vi "testIFw.vi"() -> ()   [LabVIEW 2017]
uses:
  AFE/PI_Settings.ctl
  <vilib>/rvi/Analysis/control/PID/Typedef/niFpgaPID_PIGains.ctl
  <vilib>/rvi/Analysis/control/PID/Typedef/niFpgaPID_OutputRange.ctl
  AFE/Parameters.ctl
  AFE/Mode.ctl
  <instrlib>/_niInstr/FIFO Register Bus/v1/Host/niInstr FIFO Register Bus v1 Host.lvclass
  C:/Program Files (x86)/National Instruments/LabVIEW 2017/instr.lib/_niInstr/Instruction Framework/v1/Host/Instruction Target/niInstr Instruction Target v1 Host.lvclass
  <vilib>/FPGAPlugInAG/sbRIO-9607/niLvFpga_Open_sbRIO-9607.vi
  <vilib>/rvi/interface/common/dynamic/niFpgaDynamicAddResources.vi
  <vilib>/FPGAPlugInAG/Dynamic/niLvFpga_Reset_Dynamic.vi
  <vilib>/FPGAPlugInAG/Dynamic/niLvFpga_Run_Dynamic.vi
  <vilib>/Utility/error.llb/Error Cluster From Error Code.vi
  <vilib>/rvi/errors/niLvFpgaAdjustHostInterfaceError.vi
  <vilib>/FPGAPlugInAG/Dynamic/niLvFpga_Close_Dynamic.vi
  <vilib>/rvi/interface/nirviOpenFPGA/nirviOpenFPGA.xnode
  FPGA Bitfiles/AFE_FPGATarget_IFwTest_t2qLRm+eTm8.lvbitx
  IFwTest.vi
  <vilib>/rvi/interface/nirviMethod/nirviMethod.xnode
  <vilib>/rvi/interface/nirviReadWriteControl/nirviReadWriteControl.xnode
  <vilib>/rvi/interface/nirviCloseFPGA/nirviCloseFPGA.xnode
  AFE_Interface/AFE_interface.lvlib
  AFE/ActiveFrontEnd.lvlib
  NiFpgaLv.dll
  <vilib>/rvi/interface/Simulation/niFpgaSimulationCallBeginRW.vi
panel:
  in  "IQ_to_VQ":T1={"gains"={"proportional gain"=11.0, "integral gain"=12.0}, "output range"={"output high (Inf)"=13.0, "output low (-Inf)"=14.0}, "PI_state"=enum."perturbance", "reset"=TRUE, "manual"=15.0} {"gains"."proportional gain" step=0.125}
  in  "ID_to_VD":T1={"gains"={"proportional gain"=6.0, "integral gain"=7.0}, "output range"={"output high (Inf)"=8.0, "output low (-Inf)"=9.0}, "PI_state"=enum."manual", "reset"=TRUE, "manual"=10.0} {"gains"."proportional gain" step=0.125}
  in  "VDCLinkToPower":T1={"gains"={"proportional gain"=1.0, "integral gain"=2.0}, "output range"={"output high (Inf)"=3.0, "output low (-Inf)"=4.0}, "PI_state"=enum."normal", "reset"=TRUE, "manual"=5.0} {"gains"."proportional gain" step=0.125}
  out "IQ_to_VQ_PISettings":T4
  out "ID_to_VD_PISettings":T4
  out "VDCLinkToP_PISettings":T4
  out "Parameters":T5
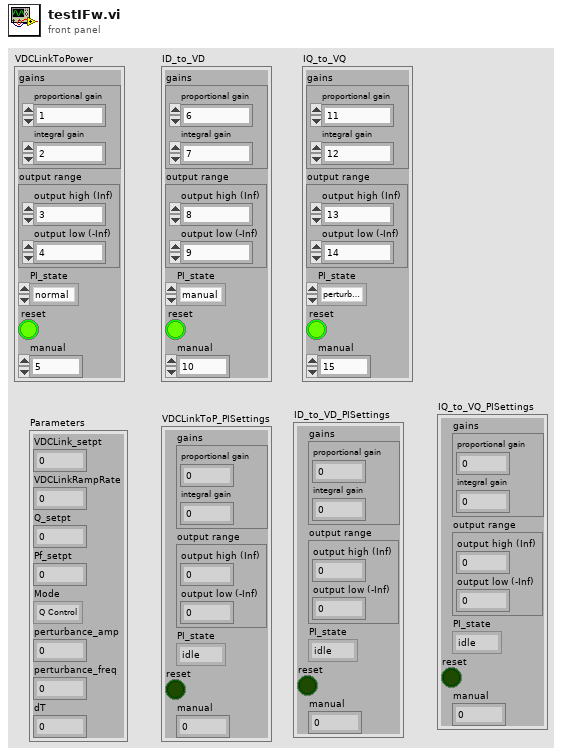
[diagram p1: front panel]
types:
  T1 = typedef "ActiveFrontEnd.lvlib/PI_Settings.ctl" = cluster{"gains":T2, "output range":T3, "PI_state":enum8{"idle", "normal", "manual", "perturbance"}, "reset":bool, "manual":sgl}
  T2 = typedef "niFpgaPID_PIGains.ctl" = cluster{"proportional gain":sgl, "integral gain":sgl}
  T3 = typedef "niFpgaPID_OutputRange.ctl" = cluster{"output high (Inf)":sgl, "output low (-Inf)":sgl}
  T4 = cluster{"gains":cluster{"proportional gain":sgl, "integral gain":sgl}, "output range":cluster{"output high (Inf)":sgl, "output low (-Inf)":sgl}, "PI_state":enum8{"idle", "normal", "manual", "perturbance"}, "reset":bool, "manual":sgl}
  T5 = cluster{"VDCLink_setpt":sgl, "VDCLinkRampRate":sgl, "Q_setpt":sgl, "Pf_setpt":sgl, "Mode":enum16{"Q Control", "Pf Control"}, "perturbance_amp":sgl, "perturbance_freq":sgl, "dT":sgl}
  T6 = typedef "ActiveFrontEnd.lvlib/Parameters.ctl" = cluster{"VDCLink_setpt":sgl, "VDCLinkRampRate":sgl, "Q_setpt":sgl, "Pf_setpt":sgl, "Mode":T7, "perturbance_amp":sgl, "perturbance_freq":sgl, "dT":sgl}
  T7 = typedef "ActiveFrontEnd.lvlib/Mode.ctl" = enum16{"Q Control", "Pf Control"}
  T8 = typedef "AFE_interface.lvlib/InterfaceRef.ctl" = cluster{"instruction target":refnum<class "niInstr Instruction Target v1 Host.lvclass">, "context":refnum<class "niInstr Instruction Framework Context v1 Host.lvclass">}
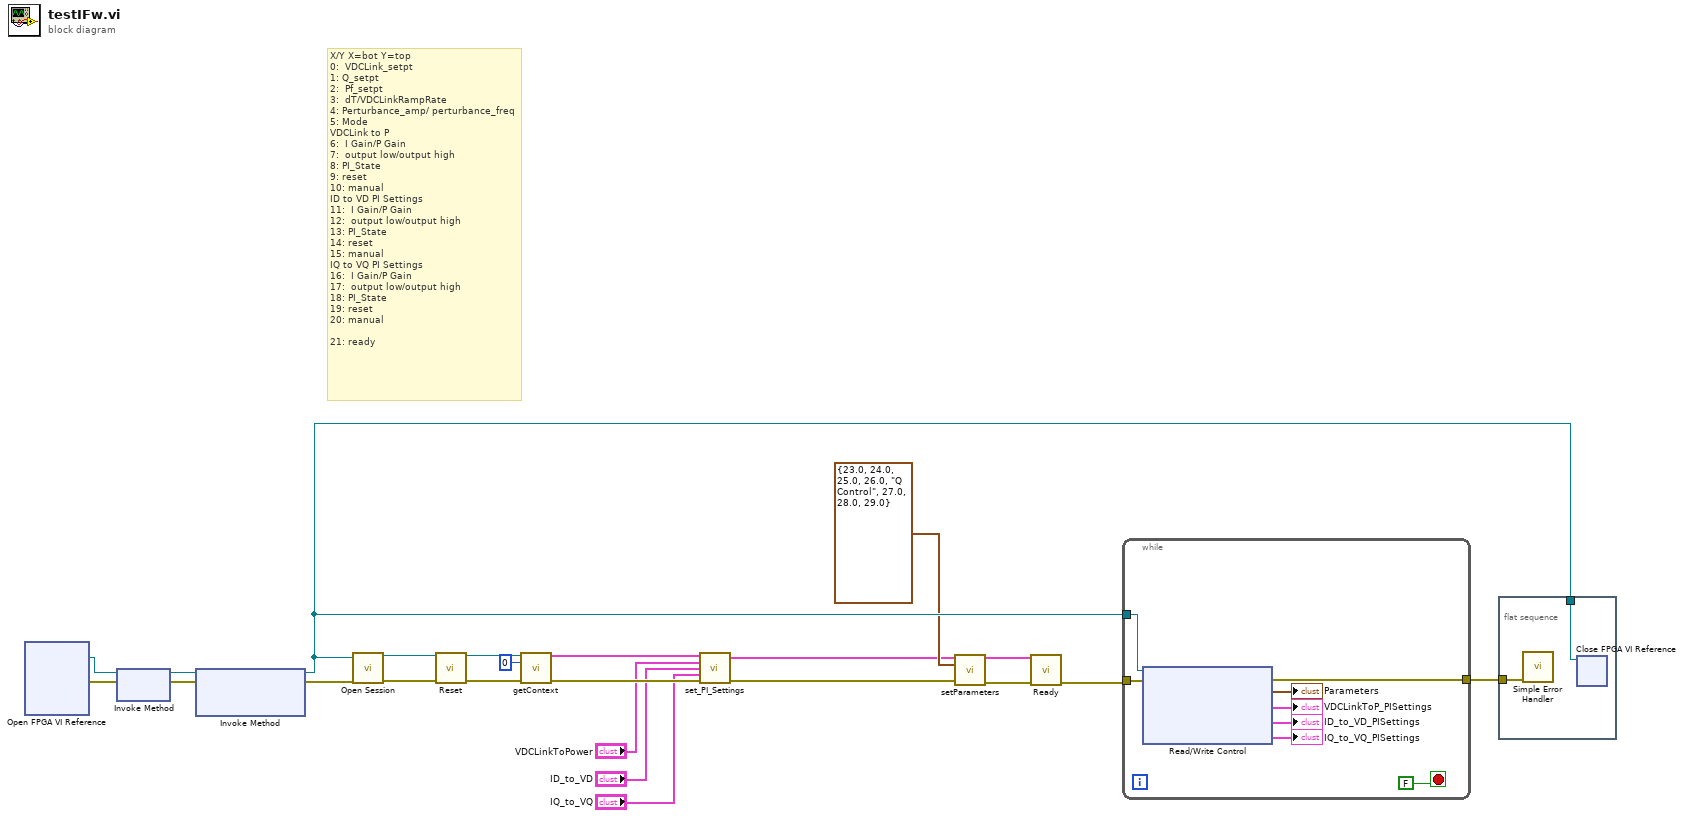
[diagram p0: block diagram]
diagram:
  # "X/Y X=bot Y=top\n0:  VDCLink_setpt\n1: Q_setpt\n2:  Pf_setpt\n3:  dT/VDCLinkRampRate\n4: Perturbance_amp/ perturbance_freq\n5: Mode\nVDCLink to P\n6:  I Gain/P Gain\n7:  output low/output high\n8: PI_State\n9: reset\n10: manual\nID to VD PI Settings \n11:  I Gain/P Gain\n12:  output low/output high\n13: PI_State\n14: reset\n15: manual\nIQ to VQ PI Settings\n16:  I Gain/P Gain\n17:  output low/output high\n18: PI_State\n19: reset\n20: manual\n\n21: ready"
  n1 = xnode "Open FPGA VI Reference"() -> ("FPGA VI Reference Out"=w17:refnum<k20>, "error out"=w16:errorcluster)  [unwired: 2 in]
  n2 = xnode "Invoke Method"("FPGA VI Reference In"=w17, "error in"=w16) -> ("FPGA VI Reference Out"=w15:refnum<k20>, "error out"=w14:errorcluster)
  n3 = xnode "Invoke Method"("FPGA VI Reference In"=w15, "error in"=w14) -> ("FPGA VI Reference Out"=w13:refnum<k20>, "error out"=w12:errorcluster)  [unwired: 1 in]
  n4 = call <instrlib>:"Open Session.vi"("fpga ref"=w13, "error in"=w12) -> ("session out"=w22:refnum<class "niInstr FIFO Register Bus v1 Host.lvclass">, "error out"=w23:errorcluster)  [unwired: 12 in]
  n5 = call-dynamic "Reset.vi"("session in"=w22, "error in"=w23) -> ("session out"=w21:refnum<class "niInstr FIFO Register Bus v1 Host.lvclass">, "error out"=w20:errorcluster)  [unwired: 12 in]
  n6 = call "getContext.vi"("instruction target in"=w21, "instance"=u8 0, "error in"=w20) -> ("Interface"=w7:T8, "error out"=w6:errorcluster)  [unwired: 11 in]
  n7 = call "set_PI_Settings.vi"("Interface in"=w7, "VDCLinkToPower"="VDCLinkToPower", "ID_to_VD"="ID_to_VD", "IQ_to_VQ"="IQ_to_VQ", "error in"=w6) -> ("Interface out"=w4:T8, "error out"=w5:errorcluster)  [unwired: 9 in]
  n8 = call "setParameters.vi"("Interface in"=w4, "Parameters"=T6 {"VDCLink_setpt"=23.0, "VDCLinkRampRate"=24.0, "Q_setpt"=25.0, "Pf_setpt"=26.0, "Mode"=enum."Q Control", "perturbance_amp"=27.0, "perturbance_freq"=28.0, "dT"=29.0}, "error in"=w5) -> ("Interface out"=w8:T8, "error out"=w10:errorcluster)  [unwired: 11 in]
  n9 = call "Ready.vi"("Interface in"=w8, "error in"=w10) -> ("error out"=w9:errorcluster)  [unwired: 12 in, 1 out]
  n10 = while {
    tunnel: w13 -> [w31]
    tunnel: w9 -> [w30]
    tunnel: [w28] -> w18
    stop <- FALSE stop-if-true
    n11 = xnode "Read/Write Control"("FPGA VI Reference In"=w31, "error in"=w30) -> ("error out"=w28:errorcluster, "Parameters"=→"Parameters":T5, "VDCLinkToP_PISettings"=→"VDCLinkToP_PISettings":T4, "ID_to_VD_PISettings"=→"ID_to_VD_PISettings":T4, "IQ_to_VQ_PISettings"=→"IQ_to_VQ_PISettings":T4)  [unwired: 1 out]
  }
  n12 = flat-sequence {
    tunnel: w18 -> [w32]
    tunnel: w13 -> [w33]
    frame #0 {
      n13 = call <vilib>:"Simple Error Handler.vi"("error in (no error)"=w32) -> ()  [unwired: 4 in, 5 out]
      n14 = xnode "Close FPGA VI Reference"("FPGA VI Reference In"=w33) -> ()  [unwired: 1 in, 1 out]
    }
  }
